vi "test_labview2_plotData.vi"() -> (3 "standard output":string)   [LabVIEW 2014]
panel:
  out "x-y":dbl
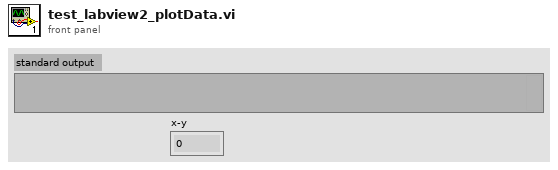
[diagram p1: front panel]
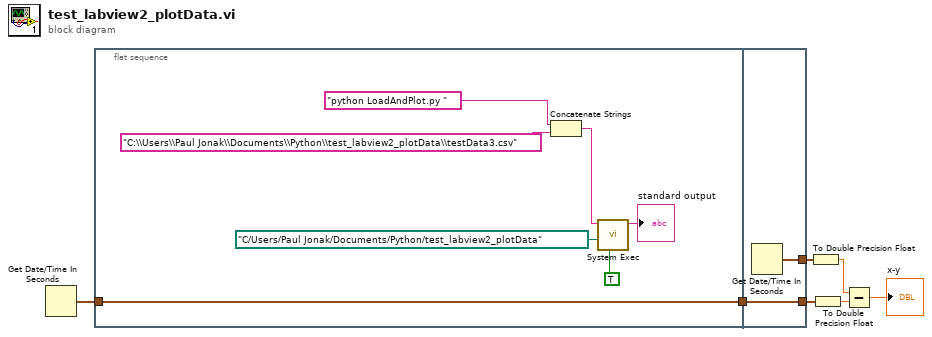
[diagram p0: block diagram]
diagram:
  n1 = Get Date/Time In Seconds() -> (seconds since 1Jan1904=w7:timestamp)
  n2 = flat-sequence {
    tunnel: w7 -> [w9]
    tunnel: [w9] -> w6
    tunnel: [w16] -> w4
    tunnel: w6 -> [w16]
    tunnel: [w15] -> w5
    frame #0 {
      n3 = Concatenate Strings("python LoadAndPlot.py " ("command line"), "C:\\Users\\Paul Jonak\\Documents\\Python\\test_labview2_plotData\\testData3.csv") -> (w11:string)
      n4 = call <vilib>:"System Exec.vi"("run minimized? (F)"=TRUE, "working directory"=path "C:/Users/Paul Jonak/Documents/Python/test_labview2_plotData", "command line"=w11) -> ("standard output"=→"standard output":string)  [unwired: 5 in, 3 out]
    }
    frame #1 {
      n5 = Get Date/Time In Seconds() -> (seconds since 1Jan1904=w15:timestamp)
    }
  }
  n6 = To Double Precision Float(number=w5) -> (double precision float=w2:dbl)
  n7 = To Double Precision Float(number=w4) -> (double precision float=w3:dbl)
  n8 = Subtract(x=w2, y=w3) -> (x-y=→"x-y":dbl)
